vi "TypeDescriptor_GetArrayElementTypeDescriptor.vi"(11 "Array Type Descriptor":i16[](array[numeric]) format="%04x") -> (1 "Element Type Descriptor":i16[](array[numeric]), 3 "Array Type Descriptor dup":i16[](array[numeric]) format="%.0x")   [LabVIEW 2013, in "OpenDescriptor.lvlib"]
uses:
  OpenDescriptor.lvlib
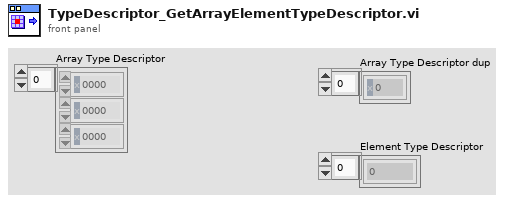
[diagram p1: front panel]
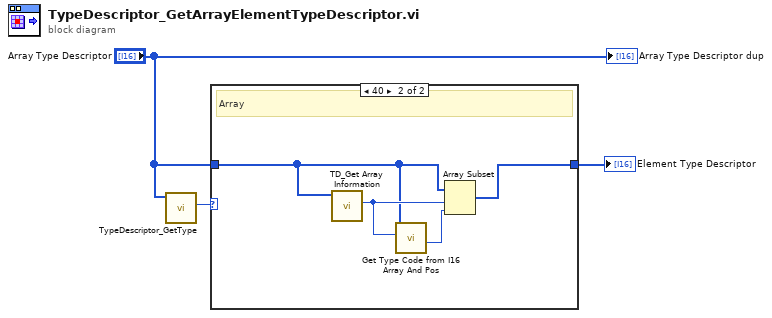
[diagram p0: block diagram]
diagram:
  n1 = call "TypeDescriptor_GetType.vi"("type descriptor"="Array Type Descriptor") -> ("Type"=w2:u8)  [unwired: 9 in, 1 out]
  n2 = case shown="40" w2 {
    tunnel: "Array Type Descriptor" -> [_ w5]
    tunnel: [_ w4] -> w1
    frame Default {
      # "Not an array"
    }
    frame 64 {
      # "Array"
      n3 = call <vilib>:"TD_Get Array Information.vi"("Type descriptor"=w5) -> ("Contained TD Offset"=w6:i32)  [unwired: 8 in, 2 out]
      n4 = call <vilib>:"Get Type Code from I16 Array And Pos.vi"("Pos in Type Descriptor (0)"=w6, "Type descriptor"=w5) -> ("Size (Words)"=w7:i32)  [unwired: 7 in, 2 out]
      n5 = Array Subset(array=w5, index=w6, length=w7) -> (w4:i16[])
    }
  }
  "Element Type Descriptor" <- w1
  "Array Type Descriptor dup" <- "Array Type Descriptor"
